vi "CloseFile.vi"(8 "error in (no error)":errorcluster, 11 "RWFile in":refnum<class "RWFile.lvclass">) -> (0 "error out":errorcluster)   [LabVIEW 2021, in "RWFile.lvclass"]
uses:
  RWFile.lvclass
  RWFile.lvclass/RWFile.ctl
  File/File.lvclass
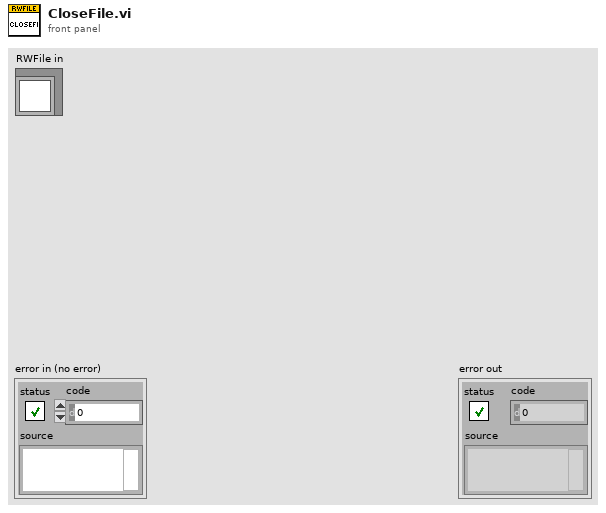
[diagram p1: front panel]
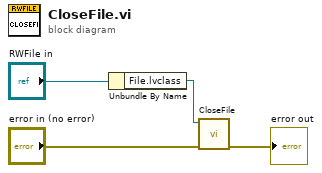
[diagram p0: block diagram]
diagram:
  n1 = Unbundle By Name("RWFile in") -> ("File.lvclass"=w1:refnum<class "File.lvclass">)
  n2 = call "CloseFile.vi"("error in (no error)"="error in (no error)", "File in"=w1) -> ("error out"=→"error out":errorcluster)  [unwired: 9 in]
